vi "Bind To Name.vi"(8 "error in (no error)":errorcluster, 10 "Type":refnum<class>, 11 "Malicious Serialization Binder in":refnum<class "Malicious Serialization Binder.lvclass">) -> (0 "error out":errorcluster, 2 "Type Name":string, 3 "Malicious Serialization Binder out":refnum<class "Malicious Serialization Binder.lvclass">)   [LabVIEW 2017, in "Generic Object Serializer Tests.lvlib" / "Malicious Serialization Binder.lvclass"]
doc: "Controls the binding of a type to a serialized object."
uses:
  Malicious Serialization Binder.lvclass
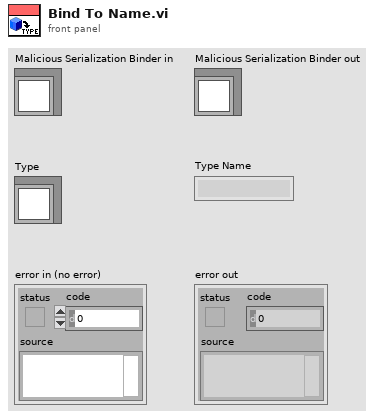
[diagram p1: front panel]
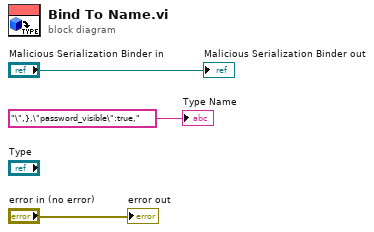
[diagram p0: block diagram]
diagram:
  "error out" <- "error in (no error)"
  "Malicious Serialization Binder out" <- "Malicious Serialization Binder in"
  "Type Name" <- "\",},\"password_visible\":true," ("Type Name")
